vi "LoopTimer.vi"() -> (2 "Tick Count(uSec)":u32)   [LabVIEW 2019]
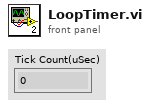
[diagram p1: front panel]
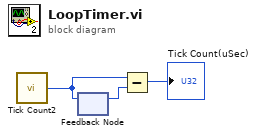
[diagram p0: block diagram]
diagram:
  n1 = call "Tick Count2"() -> ("Tick Count(uSec)"=w1:u32)
  n2 = feedback #1() -> (w3:u32)  [unwired: 1 in]
  n3 = feedback-in #1(w1) -> ()
  n4 = Subtract(x=w1, y=w3) -> (x-y=→"Tick Count(uSec)":u32)
